vi "MatFIle - Close.vi"(4 "error in":errorcluster) -> (0 "error out":errorcluster, 1 "NaN/Path/Refnum?":bool)   [LabVIEW 2023]
uses:
  controls/Action Enum.ctl
  <vilib>/Platform/storage/Storage.llb/Get Object Info.vi
  <vilib>/Platform/storage/Storage.llb/__closeStorageFromObject.vi
  <vilib>/Platform/storage/lvStorage.llb/xStorage/xStorageSupp/ErrorOut.vi
  <vilib>/Platform/storage/lvStorage.llb/xStorage/Close Data Storage/Close Data Storage.xnode
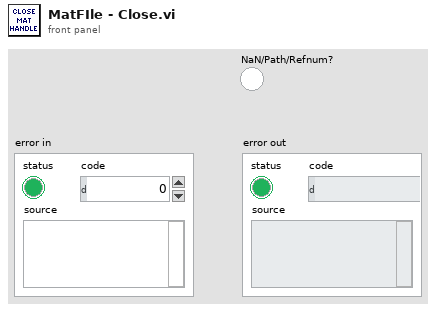
[diagram p1: front panel]
types:
  T1 = typedef "Action Enum.ctl" = enum16{"GET", "SET", "RESET"}
  T2 = enum16{"UPDATE", "READ", "QUERY", "CREATE CHILD", "CREATE", "CONNECT", "DISCONNECT"}
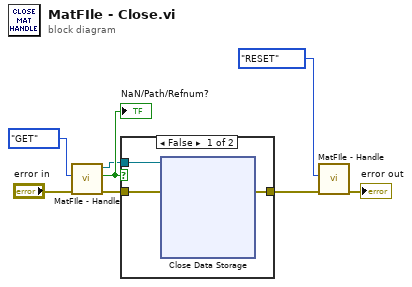
[diagram p0: block diagram]
diagram:
  n1 = call "MatFIle - Handle.vi"("error in"="error in", "Action Enum"=Action_Enum."GET") -> ("error out"=w4:errorcluster, "NaN/Path/Refnum?"=w6:bool, "storage refnum (file) out"=w5:refnum<k20>)  [unwired: 3 in]
  "NaN/Path/Refnum?" <- w6
  n2 = case shown="False" w6 {
    tunnel: w5 -> [w11 _]
    tunnel: w4 -> [w10 w20]
    tunnel: [w9 w20] -> w2
    frame False {
      n3 = xnode "Close Data Storage\n"("storage refnum (file)"=w11, "error in (no error)"=w10) -> ("error out"=w9:errorcluster)  [unwired: 1 out]
    }
    frame True {
    }
  }
  n4 = call "MatFIle - Handle.vi"("error in"=w2, "Action Enum"=Action_Enum."RESET") -> ("error out"=→"error out":errorcluster)  [unwired: 3 in, 2 out]
